vi "Sxx Measurements to Capacitance_RCV.vi"(7 "Sweep Frequency Start":dbl, 8 "error in (no error)":errorcluster, 11 "Sxx Data":cdb[](array[numeric])) -> (0 "error out":errorcluster, 3 "Capacitance":dbl[](array[numeric]))   [LabVIEW 2013]
doc: "Converts the raw S11 data from niVNA fetch into capacitance measurement."
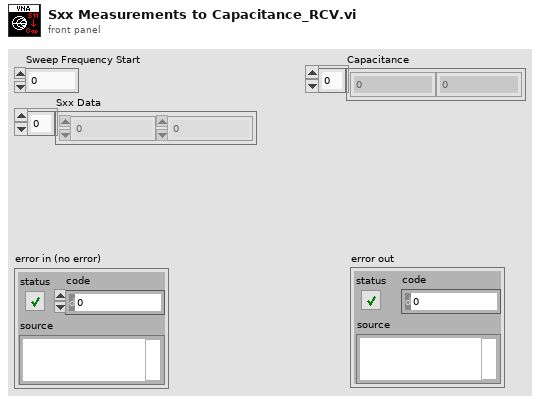
[diagram p1: front panel]
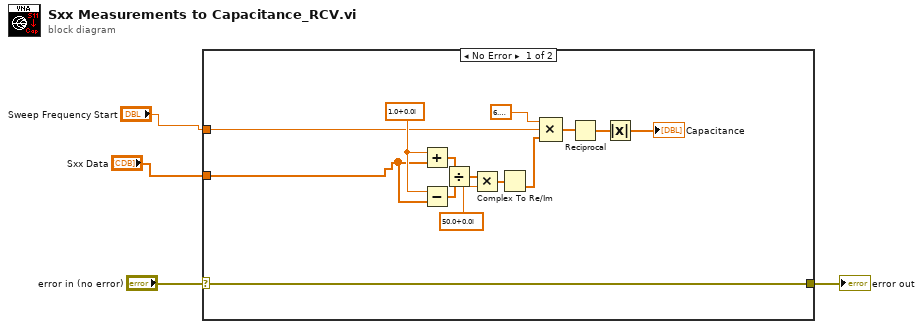
[diagram p0: block diagram]
diagram:
  n1 = case shown="No Error" "error in (no error)" {
    selector: "error in (no error)" -> [w9 w19]
    tunnel: [w9 w19] -> w4
    tunnel: "Sxx Data" -> [w8 _]
    tunnel: "Sweep Frequency Start" -> [w7 _]
    frame No Error {
      w18 = cdb 1.0+0.0i
      n2 = Add(x=w18, y=w8) -> (x+y=w17:cdb[])
      n3 = Subtract(x=w18, y=w8) -> (x-y=w16:cdb[])
      n4 = Divide(x=w17, y=w16) -> (x/y=w15:cdb[])
      n5 = Multiply(x=w15, y=cdb 50.0+0.0i) -> (x*y=w13:cdb[])
      n6 = Complex To Re/Im(x + iy=w13) -> (y=w10:dbl[])  [unwired: 1 out]
      n7 = Compound Arithmetic op=MULTIPLY(6.283185307179586, w7, w10) -> (w11:dbl[])
      n8 = Reciprocal(x=w11) -> (1/x=w6:dbl[])
      n9 = Absolute Value(x=w6) -> (abs(x)=→"Capacitance":dbl[])
    }
    frame Error {
    }
  }
  "error out" <- w4
